vi "SerialRead.vi"(8 "error in (no error)":errorcluster caption="错误输入（无错误）", 11 "serial 输入":refnum<class "serial.lvclass">) -> (0 "error out":errorcluster caption="错误输出", 1 "返回数":u32, 2 "读取反馈":string, 3 "serial 输出":refnum<class "serial.lvclass">)   [LabVIEW 2019, in "serial.lvclass"]
uses:
  serial.lvclass
  serial.lvclass/serial.ctl
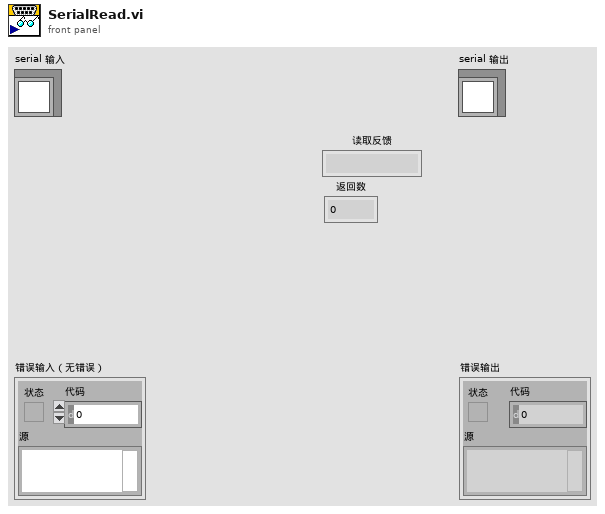
[diagram p1: front panel]
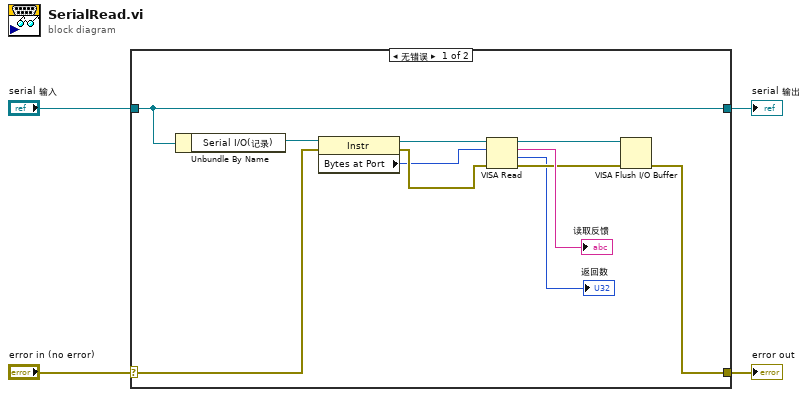
[diagram p0: block diagram]
diagram:
  n1 = case shown="无错误" "error in (no error)" {
    selector: "error in (no error)" -> [w12 w17]
    tunnel: [w5 w17] -> w3
    tunnel: [w15 w16] -> w1
    tunnel: "serial 输入" -> [w15 w16]
    frame No Error {
      n2 = Unbundle By Name(w15) -> ("Serial I/O(记录)"=w14:refnum<visa-resource-name>)
      n3 = property class="Instr"(reference=w14, error in=w12) -> (reference out=w13:refnum<visa-resource-name>, error out=w11:errorcluster, "Bytes at Port"=w10:u32)
      n4 = VISA Read(VISA resource name=w13, byte count=w10, error in (no error)=w11) -> (VISA resource name out=w8:refnum<visa-resource-name>, read buffer=→"读取反馈":string, return count=→"返回数":u32, error out=w7:errorcluster)
      n5 = VISA Flush I/O Buffer(VISA resource name=w8, error in (no error)=w7) -> (error out=w5:errorcluster)  [unwired: 1 in, 1 out]
    }
    frame Error {
    }
  }
  "error out" <- w3
  "serial 输出" <- w1
